vi "Remove Image Destination Spaces.vi"(8 "Error In":errorcluster, 11 "Images Destination In":path=path "") -> (0 "Error Out":errorcluster, 3 "Images Destination Out":path)   [LabVIEW 2018, in "Scripts.lvlib"]
uses:
  Scripts.lvlib
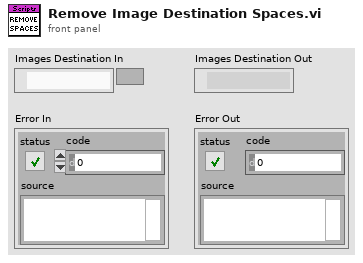
[diagram p1: front panel]
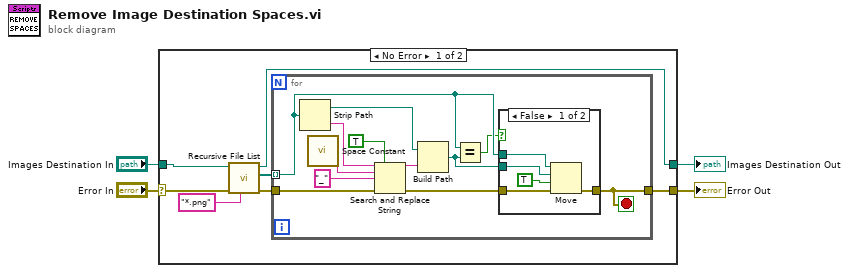
[diagram p0: block diagram]
diagram:
  n1 = case shown="No Error" "Error In" {
    selector: "Error In" -> [w7 w31]
    tunnel: [w11 w31] -> w4
    tunnel: "Images Destination In" -> [w8 w30]
    tunnel: [w6 w30] -> w1
    frame No Error {
      n2 = call <vilib>:"Recursive File List.vi"("pattern"="*.png", "error in (no error)"=w7, "Folder Path"=w8) -> ("error out"=w10:errorcluster, "All Files in Dir"=w9:path[], "dup Folder Path"=w6:path)  [unwired: 4 in, 2 out]
      n3 = for {
        tunnel: w9 -> [w15] mode=indexing
        tunnel: w10 -> [w21]
        tunnel: [w17] -> w11
        stop <- w17 stop-if-true
        n4 = Strip Path(path=w15) -> (stripped path=w19:path, name=w16:string)
        n5 = call <vilib>:"Space Constant.vi"() -> ("String"=w22:string)
        n6 = Search and Replace String(replace all?=TRUE ("replace all? (F)"), input string=w16, search string=w22, replace string="_" ("replace string (\"\")"), error in=w21) -> (result string=w18:string, error out=w20:errorcluster)  [unwired: 3 in, 2 out]
        n7 = Build Path(base path=w19, name or relative path=w18) -> (appended path=w14:path)
        n8 = Equal?(x=w15, y=w14) -> (x = y?=w13:bool)
        n9 = case shown="False" w13 {
          tunnel: w20 -> [w28 w29]
          tunnel: [w27 w29] -> w17
          tunnel: w15 -> [w26 _]
          tunnel: w14 -> [w25 _]
          frame False {
            n10 = Move(source path=w26, error in=w28, 9:TRUE ("overwrite (F)"), 10:w25) -> (error out=w27:errorcluster)  [unwired: 1 in, 2 out]
          }
          frame True {
          }
        }
      }
    }
    frame Error {
    }
  }
  "Error Out" <- w4
  "Images Destination Out" <- w1
